vi "2. Window Positioning.vi"() -> ()   [LabVIEW 2017, in "1. Basic Panels.lvlib"]
doc: "Window Positioning Example.\n----\nCopyright: MGI 2017\nAuthor: Derek Trepanier"
uses:
  1. Basic Panels.lvlib
  panel-manager/Source/Window Position/Reference Position/Alignment.ctl
  panel-manager/Source/Window Position/Reference Position/Horizontal Alignment.ctl
  panel-manager/Source/Window Position/Reference Position/Vertical Alignment.ctl
  panel-manager/Source/Window Position/Reference Position/Size/Size.lvclass
  panel-manager/Source/Window Position/Reference Position/Size/Absolute Size/Absolute Size.lvclass/Absolute Size.ctl
  panel-manager/Source/Window Position/Reference Position/Size/Reference Size/Reference Size.lvclass/Reference Size.ctl
  panel-manager/Source/Window Position/Reference Position/Size/Auto-Stretch/Auto-Stretch.lvclass/Auto-Stretch.ctl
  panel-manager/Source/Window Position/Reference Position/Offset/Absolute Offset/Absolute Offset.lvclass/Absolute Offset.ctl
  panel-manager/Source/Window Position/Reference Position/Offset/Cascade/Cascade.lvclass/Cascade.ctl
  panel-manager/Source/Window Position/Reference Position/Size/Absolute Size/Absolute Size.vi
  panel-manager/Source/Window Position/Reference Position/Size/Absolute Size/Min Panel Size.vi
  panel-manager/Source/Window Position/Reference Position/Size/Reference Size/Reference Size.vi
  panel-manager/Source/Window Position/Reference Position/Size/Auto-Stretch/Auto-Stretch.vi
  panel-manager/Source/Window Position/Reference Position/Offset/Absolute Offset/No Offset.vi
  panel-manager/Source/Window Position/Reference Position/Offset/Absolute Offset/Absolute Offset.vi
  panel-manager/Source/Window Position/Reference Position/Offset/Cascade/Cascade.vi
  panel-manager/Source/Window Position/Maximize/Maximize.vi
  panel-manager/Source/Panel/Subpanel/Subpanel.lvclass
  D:/software/LabView_PanelManager/panel-manager/Source/Panel/Panel.lvclass
  panel-manager/Source/Window Position/Reference Position/Offset/Absolute Offset/Absolute Offset.lvclass
  D:/software/LabView_PanelManager/panel-manager/Source/Window Position/Reference Position/Offset/Offset.lvclass
  panel-manager/Source/Window Position/Reference Position/Offset/Cascade/Cascade.lvclass
  panel-manager/Source/Window Position/Reference Position/Size/Absolute Size/Absolute Size.lvclass
  D:/software/LabView_PanelManager/panel-manager/Source/Window Position/Reference Position/Size/Size.lvclass
  panel-manager/Source/Window Position/Reference Position/Size/Reference Size/Reference Size.lvclass
  panel-manager/Source/Window Position/Reference Position/Size/Auto-Stretch/Auto-Stretch.lvclass
  panel-manager/Source/Window Position/Reference Position/Ref Top Level/Ref Top Level.lvclass
  D:/software/LabView_PanelManager/panel-manager/Source/Window Position/Window Position.lvclass
  panel-manager/Source/Window Position/Maximize/Maximize.lvclass
  panel-manager/Source/Window Position/Reference Position/Ref Display/Ref Display.lvclass
  panel-manager/Source/Window Position/Reference Position/Ref Rectangle/Ref Rectangle.lvclass
  panel-manager/Source/Window Position/Reference Position/Ref VI/Ref VI.lvclass
  panel-manager/Source/Window Position/Reference Position/Ref Ctrl/Ref Ctrl.lvclass
  panel-manager/Source/Panel/Window/Window.lvclass
  panel-manager/Source/Panel/Subpanel/Subpanel.vi
  panel-manager/Source/Window Position/Reference Position/Ref Top Level/Ref Top Level.vi
  panel-manager/Source/Window Position/Reference Position/Ref Display/Ref Display.vi
  panel-manager/Source/Window Position/Reference Position/Ref Rectangle/Ref Rectangle.vi
  panel-manager/Source/Window Position/Reference Position/Ref VI/Ref VI.vi
  panel-manager/Source/Window Position/Reference Position/Ref Ctrl/Ref Ctrl.vi
  panel-manager/Source/Window Position/Persistent Position/Persistent Position.vi
  panel-manager/Source/Panel/Window/Window.vi
  panel-manager/Source/MGI-Panel Manager.lvlib
  panel-manager/Source/Window Position/Persistent Position/Persistent Position.lvclass
  panel-manager/Source/Window Position/Window Position.lvclass
  panel-manager/Source/Window Position/Reference Position/Reference Position.lvclass
panel:
  in  "Size":T1(tab)
  in  "Height":i16
  in  "Width":i16
  in  "Horizontal Scale":dbl=1.0 format="%_3g"
  in  "Vertical Scale":dbl=1.0 format="%_3g"
  in  "Vertical?":bool=TRUE
  in  "Horizontal?":bool=TRUE
  in  "Offset":enum32{"No Offset", "Absolute", "Cascade"}(tab)
  in  "Vertical":i16
  in  "Horizontal":i16
  in  "Cascade Group":string="Default"
  in  "Vertical Step":i16=20
  in  "Horizontal Step":i16=20
  in  "Alignment":T2={"Horizontal"=enum."Center", "Vertical"=enum."Center"}
  in  "Show Window":bool
  in  "Tab Control":T5(tab)
  in  "Rectangle":T6
  in  "VI ID":string
  # "Run this VI to view the Window Positioning Example"
  # "This will not resize the VI. Whatever the last size of the Panel was will be used.\n\nNote: Inserting a VI into a subpanel changes it's size. That means that if you launch a panel as a subpanel, then later as a window, the size of the window will be the same size as your subpanel. If that is your use case then you may want to used one of the other size types.\nNote: If you're launching several clones of the same panel, then you're new panel may be a reused clone from a closed clone. This new panel will have the same size as whatever the closed clone had.  If that is your use case then you may want to use one of the other size types."
  # "This forces static a window size"
  # "This sets the window size equal to the minimum panel size of the new window."
  # "This sets the size based on the referenced item (VI, Control, Display, etc)"
  # "This panel size will automatically calculate the size based on the controls on the front panel.\n\nThe panel will be grown or shrunk appropriately to fit all of the visible controls on the front panel. This allows you to programatically position and resize controls before the panel is shown, then the panel will automatically be resized before the framework displays it."
  # "No offset is applied. The window position is based only on the aligment input."
  # "A static offset is applied."
  # "Similar windows (as specified by cascade group) are cascaded together. If the window is moved from its initial position or closed, the next window in the group will take its place."
  # "This will position the window based on the top level VI. The Panel Manager Framework will automatically determine the top level UI VI. This means that if a subpanel UI launches a window with the \"Top Level\" positioner, the new window will be positioned using owner of the subpanel's VI.\n\nNotice how the \"Show Dialog\" button in the subpanel above and the \"Show Window\" button below both center the new panel in this VI."
  # "This will position the new panel based on the active display."
  # "This will position the new window based on another VI's front panel.\n\nIn this example it will position the panel based on this VI."
  # "This will position the new window based on another control.\n\nIn this example, the \"Show Window\" button is used as the reference control."
  # "This will position the new window based on the specified rectangle."
  # "This will maximize the window.\n\nThis option ignores the Alignment, Size, and Offset inputs."
  # "This position size will remember the last position of the window between application executions. Each window's position will be saved in a file on the filesystem.\n\nThis option ignores the Alignment, Size, and Offset inputs."
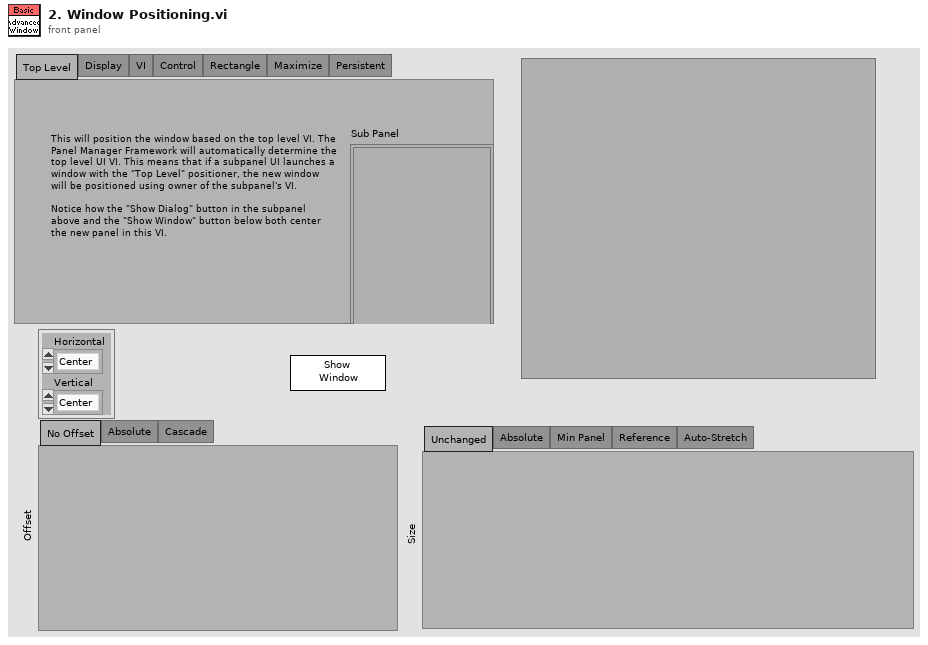
[diagram p1: front panel]
types:
  T1 = enum32{"Unchanged", "Absolute", "Min Panel", "Reference", "Auto-Stretch"}
  T2 = typedef "MGI-Panel Manager.lvlib/Reference Position.lvclass/Alignment.ctl" = cluster{"Horizontal":T3, "Vertical":T4}
  T3 = typedef "MGI-Panel Manager.lvlib/Reference Position.lvclass/Horizontal Alignment.ctl" = enum16{"Left", "Center", "Right"}
  T4 = typedef "MGI-Panel Manager.lvlib/Reference Position.lvclass/Vertical Alignment.ctl" = enum16{"Top", "Center", "Bottom"}
  T5 = enum32{"Top Level", "Display", "VI", "Control", "Rectangle", "Maximize", "Persistent"}
  T6 = cluster{"left":i16, "top":i16, "right":i16, "bottom":i16}
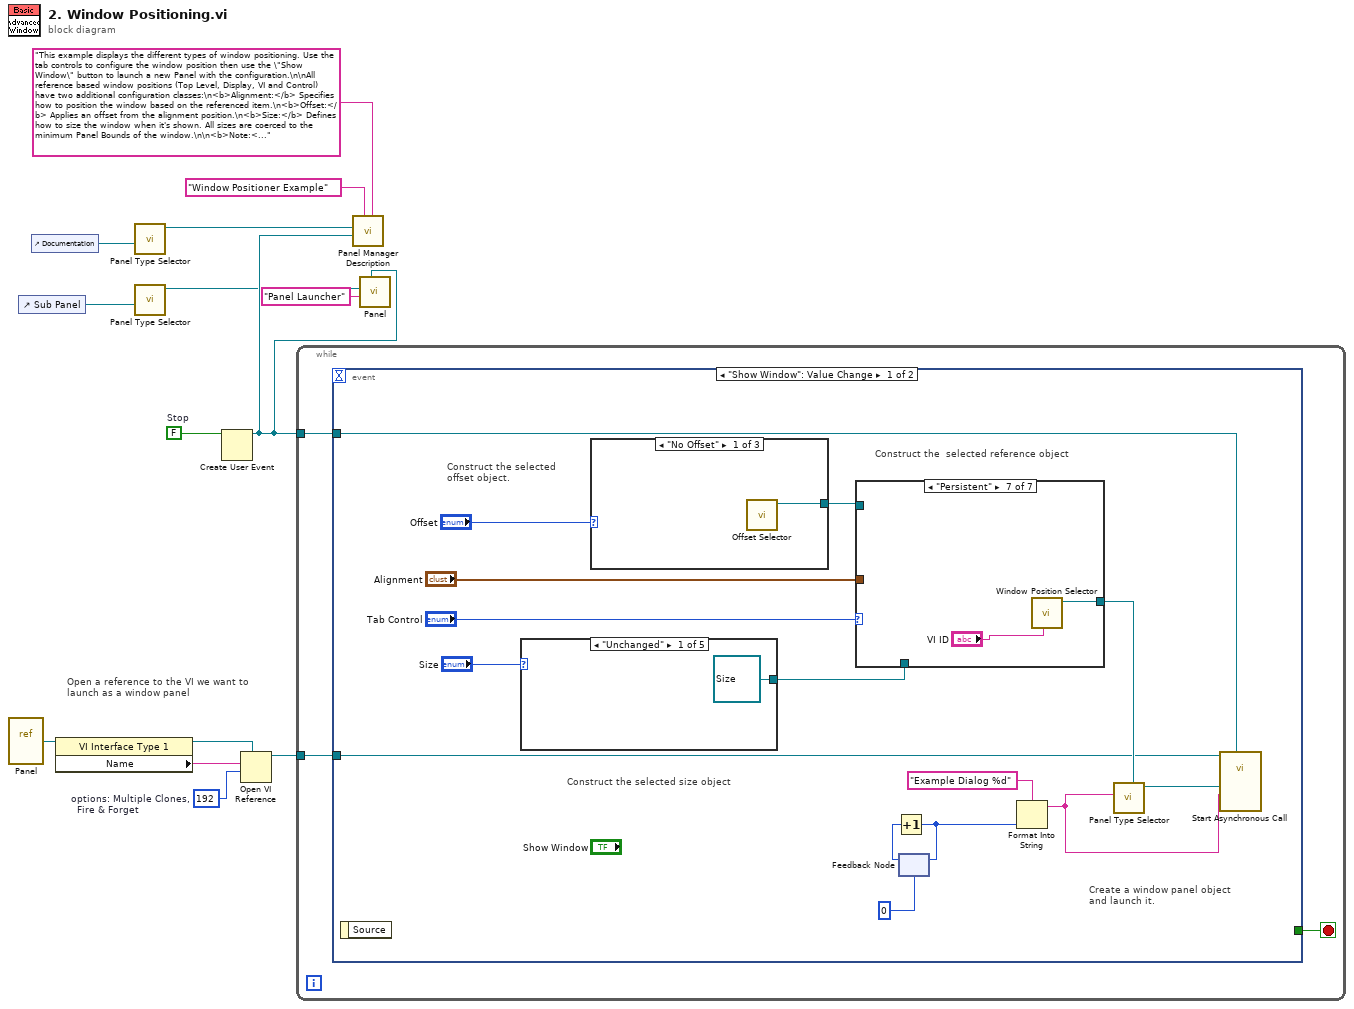
[diagram p0: block diagram]
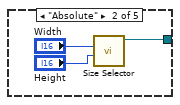
[diagram p2: hidden frame]
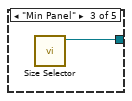
[diagram p3: hidden frame]
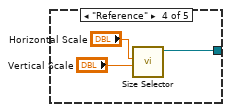
[diagram p4: hidden frame]
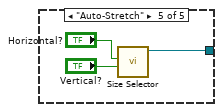
[diagram p5: hidden frame]
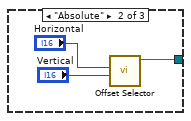
[diagram p6: hidden frame]
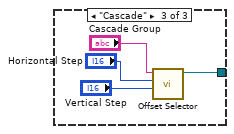
[diagram p7: hidden frame]
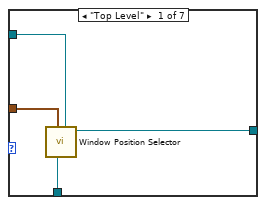
[diagram p8: hidden frame]
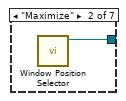
[diagram p9: hidden frame]
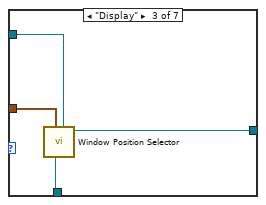
[diagram p10: hidden frame]
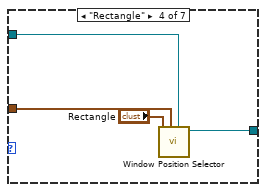
[diagram p11: hidden frame]
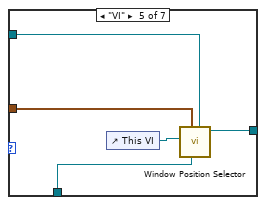
[diagram p12: hidden frame]
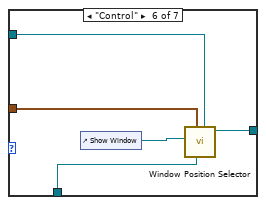
[diagram p13: hidden frame]
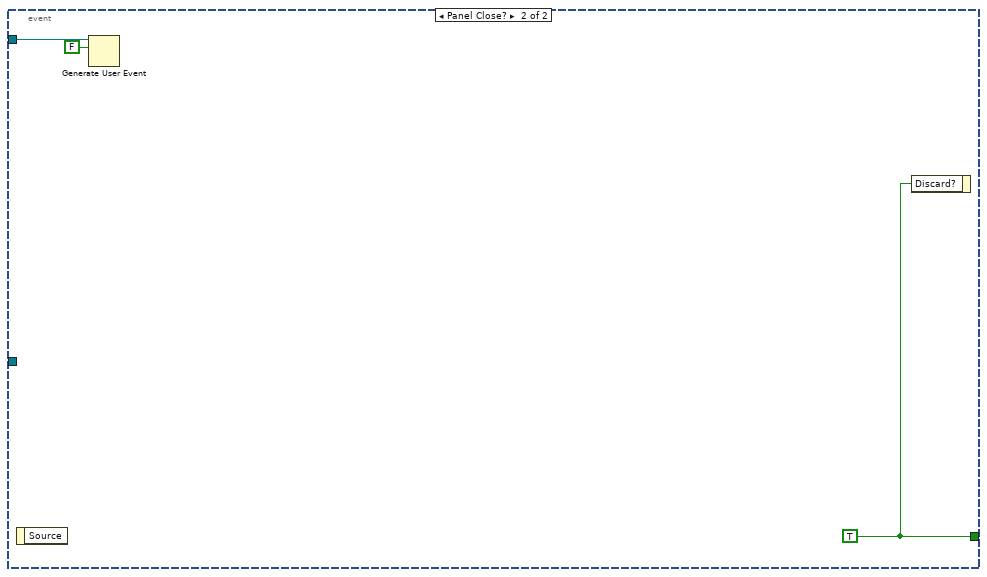
[diagram p14: hidden frame]
diagram:
  w2 = 192  # options: Multiple Clones,   Fire & Forget
  w11 = FALSE  # Stop
  # "Open a reference to the VI we want to launch as a window panel"
  n1 = vi-ref "Panel.vi"() -> (w5:refnum<vi>)
  n2 = control-ref of="Sub Panel"() -> (w9:refnum<vi>)
  n3 = control-ref of="Documentation"() -> (w13:refnum<vi>)
  n4 = property class="VI Interface Type 1"(reference=w5) -> (reference out=w4:refnum<vi>, "Name"=w3:string)  [unwired: 1 in, 1 out]
  n5 = call-poly "Panel Type Selector.vi"("Sub Panel"=w13) -> ("Subpanel Out"=w14:refnum<class "Subpanel.lvclass">)  [unwired: 9 in, 1 out]
  n6 = call-poly "Panel Type Selector.vi"("Sub Panel"=w9) -> ("Subpanel Out"=w7:refnum<class "Subpanel.lvclass">)  [unwired: 9 in, 1 out]
  n7 = Create User Event(user event datatype=w11) -> (user event=w8:refnum<user-event>)  [unwired: 1 in, 1 out]
  n8 = Open VI Reference(type specifier VI Refnum (for type only)=w4, vi path=w3, options=w2) -> (vi reference=w1:refnum<vi>)  [unwired: 3 in, 1 out]
  n9 = while {
    tunnel: w8 -> [w16]
    tunnel: w1 -> [w15]
    stop <- w17 stop-if-true
    n10 = event shown="[0] \"Show Window\": Value Change" {
      selector: _ -> [_ _]
      dyn-events: _ -> [_ _]
      timeout: _ -> [_ _]
      tunnel: [_ w77] -> w17
      tunnel: w16 -> [w25 w79]
      tunnel: w15 -> [w27 _]
      event "Show Window": Value Change {
        # "Create a window panel object\nand launch it."
        # "Construct the  selected reference object"
        # "Construct the selected\noffset object."
        # "Construct the selected size object"
        n11 = event-data() -> ()  [unwired: 1 in, 1 out]
        n12 = case shown="\"Unchanged\"" "Size" {
          tunnel: [refnum<class "Size.lvclass"> refnum ("Static out") w34 w37 w40 w43] -> w18
          frame "Unchanged" {
          }
          frame "Absolute" {
            n13 = call-poly "Size Selector.vi"("Height"="Height", "Width"="Width") -> ("Absolute Size out"=w34:refnum<class "Absolute Size.lvclass">)  [unwired: 8 in, 1 out]
          }
          frame "Min Panel" {
            n14 = call-poly "Size Selector.vi"() -> ("Static out"=w37:refnum<class "Absolute Size.lvclass">)  [unwired: 10 in, 1 out]
          }
          frame "Reference" {
            n15 = call-poly "Size Selector.vi"("Height Scale"="Vertical Scale", "Width Scale"="Horizontal Scale") -> ("Static Out"=w40:refnum<class "Reference Size.lvclass">)  [unwired: 8 in, 1 out]
          }
          frame "Auto-Stretch" {
            n16 = call-poly "Size Selector.vi"("Vertical?"="Vertical?", "Horizontal?"="Horizontal?") -> ("Auto-Stretch Out"=w43:refnum<class "Auto-Stretch.lvclass">)  [unwired: 8 in, 1 out]
          }
        }
        n17 = case shown="\"No Offset\"" "Offset" {
          tunnel: [w44 w47 w51] -> w29
          frame "No Offset" {
            n18 = call-poly "Offset Selector.vi"() -> ("Absolute Offset Out"=w44:refnum<class "Absolute Offset.lvclass">)  [unwired: 10 in, 1 out]
          }
          frame "Absolute" {
            n19 = call-poly "Offset Selector.vi"("Vertical"="Vertical", "Horizontal"="Horizontal") -> ("Absolute Offset Out"=w47:refnum<class "Absolute Offset.lvclass">)  [unwired: 8 in, 1 out]
          }
          frame "Cascade" {
            n20 = call-poly "Offset Selector.vi"("Vertical Step"="Vertical Step", "Horizontal Step"="Horizontal Step", "Cascade"="Cascade Group") -> ("Cascade out"=w51:refnum<class "Cascade.lvclass">)  [unwired: 7 in, 1 out]
          }
        }
        n21 = case shown="\"Persistent\"" "Tab Control" {
          tunnel: [w55 w56 w60 w64 w69 w74 w76] -> w32
          tunnel: "Alignment" -> [w54 _ w59 w63 w68 w73 _]
          tunnel: w29 -> [w53 _ w58 w62 w66 w72 _]
          tunnel: w18 -> [w52 _ w57 _ w65 w70 _]
          frame "Top Level" {
            n22 = call-poly "Window Position Selector.vi"("Offset"=w53, "Size"=w52, "Alignment"=w54) -> ("Ref Top Level out"=w55:refnum<class "Ref Top Level.lvclass">)  [unwired: 7 in, 1 out]
          }
          frame "Maximize" {
            n23 = call-poly "Window Position Selector.vi"() -> ("Maximize out"=w56:refnum<class "Maximize.lvclass">)  [unwired: 10 in, 1 out]
          }
          frame "Display" {
            n24 = call-poly "Window Position Selector.vi"("Offset"=w58, "Size"=w57, "Alignment"=w59) -> ("Ref Display out"=w60:refnum<class "Ref Display.lvclass">)  [unwired: 7 in, 1 out]
          }
          frame "Rectangle" {
            n25 = call-poly "Window Position Selector.vi"("Offset"=w62, "Alignment"=w63, "Rectangle"="Rectangle") -> ("Ref Rectangle"=w64:refnum<class "Ref Rectangle.lvclass">)  [unwired: 7 in, 1 out]
          }
          frame "VI" {
            n26 = control-ref of="This VI"() -> (w67:refnum<vi>)
            n27 = call-poly "Window Position Selector.vi"("Offset"=w66, "Size"=w65, "Alignment"=w68, "Ref VI"=w67) -> ("Ref VI out"=w69:refnum<class "Ref VI.lvclass">)  [unwired: 6 in, 1 out]
          }
          frame "Control" {
            n28 = control-ref of="Show Window"() -> (w71:refnum<vi>)
            n29 = call-poly "Window Position Selector.vi"("Offset"=w72, "Size"=w70, "Alignment"=w73, "Ref Ctrl"=w71) -> ("Ref Ctrl Out"=w74:refnum<class "Ref Ctrl.lvclass">)  [unwired: 6 in, 1 out]
          }
          frame "Persistent" {
            n30 = call-poly "Window Position Selector.vi"("VI ID"="VI ID") -> ("Persistent Position out"=w76:refnum<class "Window Position.lvclass">)  [unwired: 9 in, 1 out]
          }
        }
        n31 = feedback #1(0) -> (w23:i32)
        n32 = Increment(x=w23) -> (x+1=w20:i32)
        n33 = feedback-in #1(w20) -> ()
        n34 = Format Into String(format string="Example Dialog %d" ("Default Title"), w20) -> (resulting string=w21:string)  [unwired: 2 in, 1 out]
        n35 = call-poly "Panel Type Selector.vi"("Window Position"=w32, "Default Title"=w21) -> ("Window out"=w26:refnum<class "Window.lvclass">)  [unwired: 8 in, 1 out]
        n36 = call-by-ref "Start Asynchronous Call"(reference=w27, "Stop Event"=w25, "Label"=w21, "Panel"=w26) -> ()  [unwired: 10 in, 2 out]
      }
      event Panel Close? {
        w77 = TRUE
        n37 = event-data() -> ()  [unwired: 1 in, 1 out]
        n38 = Generate User Event(user event=w79, event data cluster=FALSE ("event data")) -> ()  [unwired: 2 in, 2 out]
        n39 = event-data("Discard?"=w77) -> ()  [unwired: 1 in, 1 out]
      }
    }
  }
  n40 = call "Panel Manager Description.vi"("Description"="This example displays the different types of window positioning. Use the tab controls to configure the window position then use the \"Show Window\" button to launch a new Panel with the configuration.\n\nAll reference based window positions (Top Level, Display, VI and Control) have two additional configuration classes:\n<b>Alignment:</b> Specifies how to position the window based on the referenced item.\n<b>Offset:</b> Applies an offset from the alignment position.\n<b>Size:</b> Defines how to size the window when it's shown. All sizes are coerced to the minimum Panel Bounds of the window.\n\n<b>Note:</b> The \"Window Position\" class is overridable. This means if the built-in items don't do what you need, you can implement your own window position algorithm.\n\nWindows in this example are launched as Window Panels, but the window positioning applies to both Window and Dialog Panel types.\n" ("Description Title"), "Description Title"="Window Positioner Example", "Stop Event"=w8, "Panel"=w14) -> ()  [unwired: 7 in, 1 out]
  n41 = call "Panel.vi"("Stop Event"=w8, "Label"="Panel Launcher", "Panel"=w7) -> ()  [unwired: 9 in]
